vi "Read Results from processing.vi"(8 "error in":errorcluster, 11 "ExampleSequencer runtime in":refnum<class "ExampleSequencer runtime.lvclass">) -> (0 "error out":errorcluster, 2 "Results from processing":T1, 3 "ExampleSequencer runtime out":refnum<class "ExampleSequencer runtime.lvclass">)   [LabVIEW 2017, in "ExampleSequencer runtime.lvclass"]
uses:
  ExampleSequencer runtime.lvclass
  configuration/result data indices.ctl
  ExampleSequencer runtime.lvclass/ExampleSequencer runtime.ctl
  configuration/ExampleSequencer configuration.lvclass
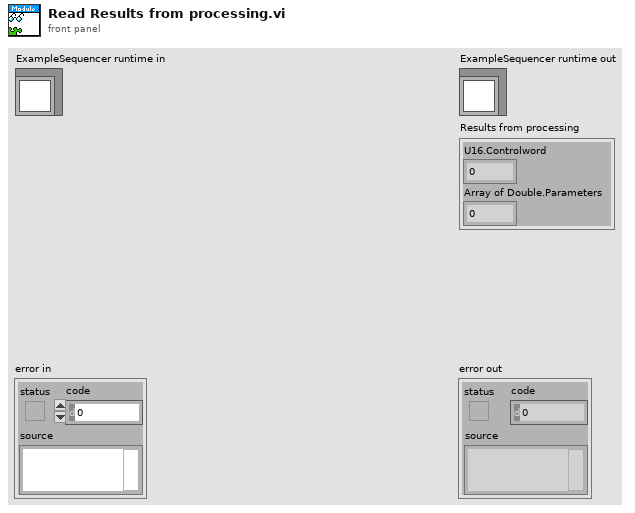
[diagram p1: front panel]
types:
  T1 = typedef "ExampleSequencer configuration.lvclass/result data indices.ctl" = cluster{"U16.Controlword":i32, "Array of Double.Parameters":i32}
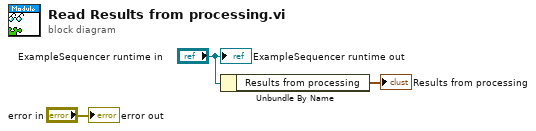
[diagram p0: block diagram]
diagram:
  n1 = Unbundle By Name("ExampleSequencer runtime in") -> ("Results from processing"=→"Results from processing":T1)
  "error out" <- "error in"
  "ExampleSequencer runtime out" <- "ExampleSequencer runtime in"
